vi "Update Default values.vi"(11 "VI in":refnum<vi>) -> (3 "Default Values out":variant[](array[variant]))   [LabVIEW 2013]
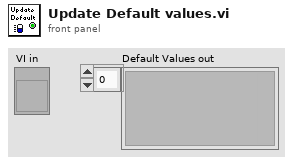
[diagram p1: front panel]
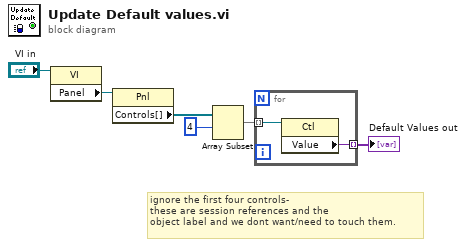
[diagram p0: block diagram]
diagram:
  # "ignore the first four controls-\nthese are session references and the\nobject label and we dont want/need to touch them."
  n1 = property class="VI"(reference="VI in") -> ("Panel"=w4:refnum<vi>)  [unwired: 1 in, 2 out]
  n2 = property class="Pnl"(reference=w4) -> ("Controls[]"=w2:refnum<vi>[])  [unwired: 1 in, 2 out]
  n3 = Array Subset(array=w2, index=4) -> (w1:refnum<vi>[])  [unwired: 1 in]
  n4 = for {
    tunnel: [w8] -> w6 mode=indexing
    tunnel: w1 -> [w7] mode=indexing
    n5 = property class="Ctl"(reference=w7) -> ("Value"=w8:variant)  [unwired: 1 in, 2 out]
  }
  "Default Values out" <- w6
